vi "RF_Synth_move.vi"(1 "Points":cluster{string, "data":u64, "data":dbl}, 2 "Instr. Info":T1) -> ()   [LabVIEW 2013]
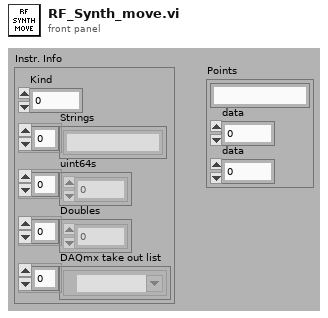
[diagram p1: front panel]
types:
  T1 = cluster{"Kind":u16, "Strings":string[], "uint64s":u64[], "Doubles":dbl[], "DAQmx take out list":refnum<k21>[]}
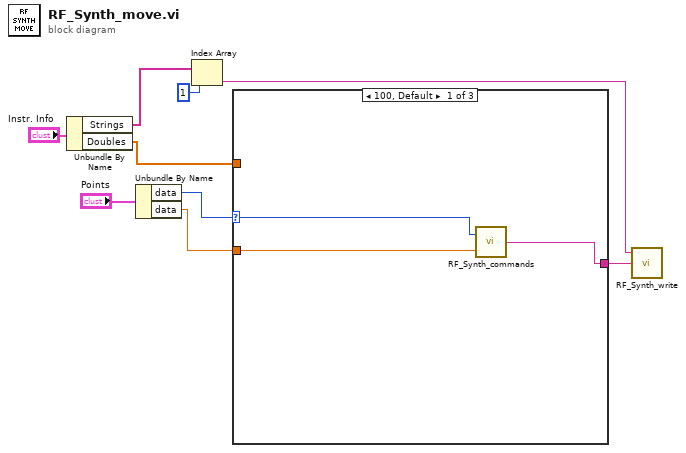
[diagram p0: block diagram]
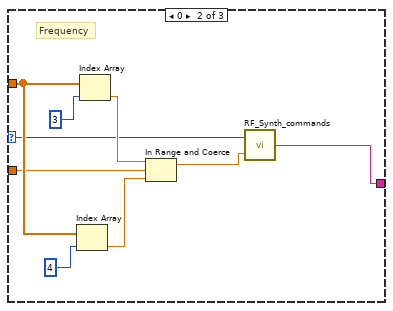
[diagram p2: hidden frame]
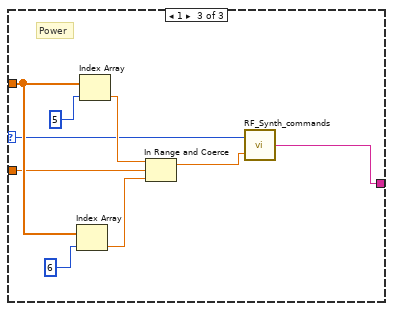
[diagram p3: hidden frame]
diagram:
  n1 = Unbundle By Name("Instr. Info") -> ("Strings"=w7:string[], "Doubles"=w4:dbl[])
  n2 = Unbundle By Name("Points") -> ("data"=w3:u64, "data"=w5:dbl)
  n3 = Index Array(array=w7, index=1) -> (element=w2:string)
  n4 = case shown="100, Default" w3 {
    selector: w3 -> [w12 w15 w24]
    tunnel: w5 -> [w11 w19 w28]
    tunnel: w4 -> [_ w21 w30]
    tunnel: [w10 w13 w22] -> w1
    frame 100, Default {
      n5 = call "RF_Synth_commands.vi"("Value"=w11, "Parameter"=w12) -> ("Command"=w10:string)
    }
    frame 0 {
      # "Frequency"
      n6 = Index Array(array=w21, index=4) -> (element=w17:dbl)
      n7 = Index Array(array=w21, index=3) -> (element=w18:dbl)
      n8 = In Range and Coerce(upper limit=w18, x=w19, lower limit=w17) -> (coerced(x)=w14:dbl)  [unwired: 1 out]
      n9 = call "RF_Synth_commands.vi"("Value"=w14, "Parameter"=w15) -> ("Command"=w13:string)
    }
    frame 1 {
      # "Power"
      n10 = Index Array(array=w30, index=6) -> (element=w26:dbl)
      n11 = Index Array(array=w30, index=5) -> (element=w27:dbl)
      n12 = In Range and Coerce(upper limit=w27, x=w28, lower limit=w26) -> (coerced(x)=w23:dbl)  [unwired: 1 out]
      n13 = call "RF_Synth_commands.vi"("Value"=w23, "Parameter"=w24) -> ("Command"=w22:string)
    }
  }
  n14 = call "RF_Synth_write.vi"("write buffer"=w1, "VISA resource name"=w2) -> ()  [unwired: 1 in, 1 out]
